vi "PID.vi"() -> ()   [LabVIEW 2019]
panel:
  in  "TURNING":cluster{"P":dbl, "I":dbl, "D":dbl}
  in  "INTAKE PIVOT":T1
  in  "SHOOTER":T1
  in  "TURRET":T1
  in  "AUTO_PID":cluster{"P":dbl, "I":dbl, "D":dbl}
  in  "PID":T1
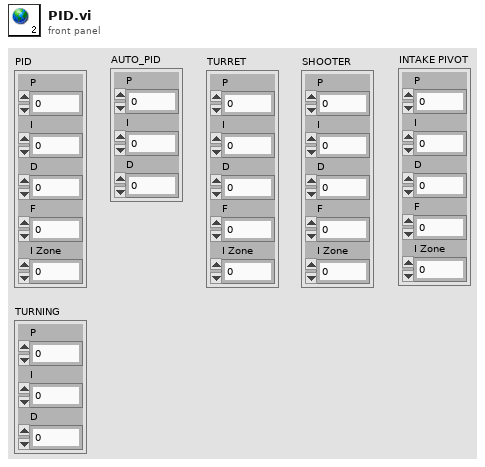
[diagram p1: front panel]
types:
  T1 = cluster{"P":dbl, "I":dbl, "D":dbl, "F":dbl, "I Zone":dbl}
diagram:
